vi "Grab and Detect Skipped Buffers.vi"() -> ()   [LabVIEW 2011]
doc: "The Grab and Detect Skipped Buffers VI acquires images continuously and displays the images in an image control using high-level acquisition VIs. The VI uses buffer number to detect missed frames. A grab is appropriate for high-speed applications in which you need to process only one image at a time."
uses:
  <vilib>/vision/driver/NI_Vision_Acquisition_Software.lvlib
  <vilib>/vision/driver/IMAQdx.llb/IMAQdx Buffer Number Mode.ctl
panel:
  in  "Camera Name":refnum<k21> caption="IMAQdx Session"
  out "Skipped Buffer Count":u32
  out "Buffer Number":u32
  out "Image":T1(plugin-control)
  out "Buffer Number Delta":u32(knob) scale=0.0..5.0
  out "Processed Frame Rate":dbl(knob) scale=0.0..100.0
  out "Acquired Frame Rate":dbl(knob) scale=0.0..100.0
  in  "Stop":bool
  # "Overview: Demonstrates how to monitor an acquisition for missed frames.\nRequirements: Vision Acquisition Software\nInstructions: \n1. Select the Camera Name.\n2. Run the VI"
  # "In an ideal system, the acquired frame rate and the processed frame rate are the same. Also, the buffer number delta from iteration to iteration is 1. If the image processing interval exceeds the acquired frame interval, the processed frame rate drops below the acquired frame rate, and the buffer number delta goes above 1. At this point, the application skips buffers. To prevent your application from  skipping buffers, reduce the amount of image processing or reduce the frame rate.\n\nNOTE: On Windows operating systems, background tasks may influence the processed frame rate."
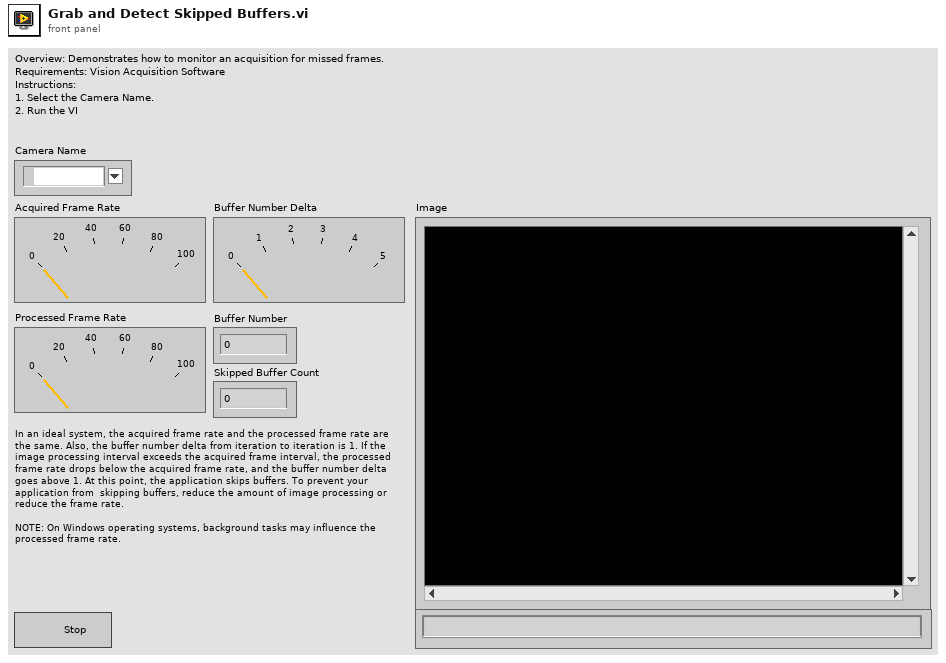
[diagram p1: front panel]
types:
  T1 = typedef "IMAQ Image.ctl" = refnum<image>
  T2 = typedef "IMAQdx.ctl" = refnum<k21>
  T3 = typedef "NI_Vision_Acquisition_Software.lvlib/IMAQdx Buffer Number Mode.ctl" = enum32{"Next", "Last", "Buffer Number", "Every", "Last New"}
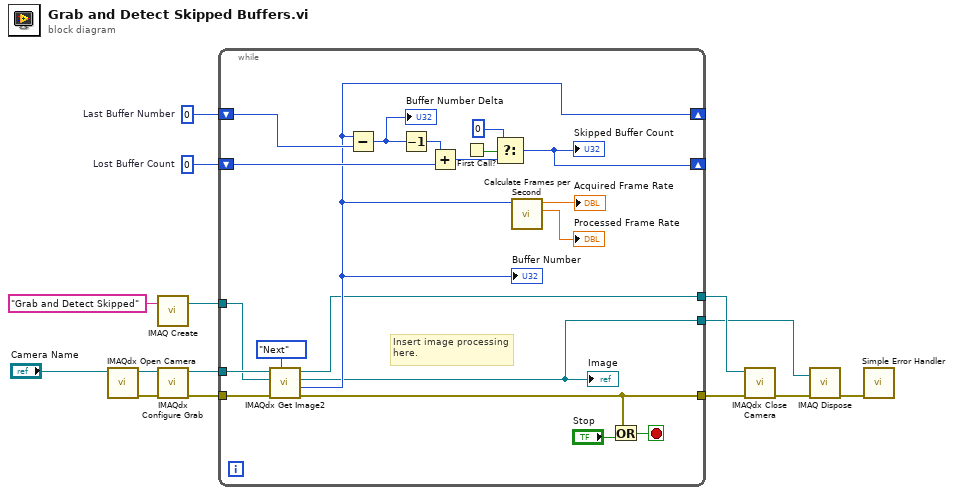
[diagram p0: block diagram]
diagram:
  w6 = u32 0  # Lost Buffer Count
  w7 = u32 0  # Last Buffer Number
  n1 = call <vilib>:"IMAQdx Open Camera.vi"("Session In"="Camera Name") -> ("error out"=w10:errorcluster, "Session Out"=w9:T2)  [unwired: 2 in, 7 out]
  n2 = call "IMAQ Create"("Image Name"="Grab and Detect Skipped") -> ("New Image"=w14:T1)  [unwired: 3 in, 2 out]
  n3 = call <vilib>:"IMAQdx Configure Grab.vi"("error in"=w10, "Session In"=w9) -> ("error out"=w12:errorcluster, "Session Out"=w13:T2)  [unwired: 8 out]
  n4 = while {
    tunnel: w12 -> [w32]
    tunnel: w13 -> [w33]
    tunnel: [w16] -> w11
    tunnel: w14 -> [w31]
    shift-right: [w18] -> _
    shift-left: w7 -> [w29]
    tunnel: [w17] -> w8
    shift-right: [w22] -> _
    shift-left: w6 -> [w28]
    tunnel: [w15] -> w3
    stop <- w34 stop-if-true
    # "Insert image processing here."
    n5 = call <vilib>:"IMAQdx Get Image2.vi"("Buffer Number Mode (Next)"=IMAQdx_Buffer_Number_Mode."Next", "error in"=w32, "Image In"=w31, "Session In"=w33) -> ("error out"=w16:errorcluster, "Buffer Number Out"=w18:u32, "Image Out"=w15:T1, "Session Out"=w17:T2)  [unwired: 4 in]
    "Image" <- w15
    "Buffer Number" <- w18
    n6 = Subtract(x=w18, y=w29) -> (x-y=w27:u32)
    "Buffer Number Delta" <- w27
    n7 = Decrement(x=w27) -> (x-1=w26:u32)
    n8 = Add(x=w26, y=w28) -> (x+y=w25:u32)
    n9 = First Call?() -> (First Call?: T/F=w24:bool)
    n10 = Select(t=u32 0, s=w24, f=w25) -> (s? t:f=w22:u32)
    "Skipped Buffer Count" <- w22
    n11 = call <vilib>:"Calculate Frames per Second.vi"("Buffer Number"=w18) -> ("Processed Frames/s"=→"Processed Frame Rate":dbl, "Acquired Frames/s"=→"Acquired Frame Rate":dbl)  [unwired: 8 in, 1 out]
    n12 = Or(x=w16, y="Stop") -> (x .or. y?=w34:bool)
  }
  n13 = call <vilib>:"IMAQdx Close Camera.vi"("error in"=w11, "Session In"=w8) -> ("error out"=w2:errorcluster)  [unwired: 9 out]
  n14 = call "IMAQ Dispose"("Image"=w3, "error in (no error)"=w2) -> ("error out"=w1:errorcluster)  [unwired: 4 in]
  n15 = call <vilib>:"Simple Error Handler.vi"("error in (no error)"=w1) -> ()  [unwired: 1 in, 8 out]
